vi "Read Directory.vi"(8 "error in (no error)":errorcluster, 11 "TreeDirectory in":refnum<class "TreeDirectoryExt.lvclass">) -> (0 "error out":errorcluster, 2 "Path":path, 3 "TreeDirectory out":refnum<class "TreeDirectoryExt.lvclass">)   [LabVIEW 2026, in "TreeDirectoryExt.lvclass"]
uses:
  TreeDirectoryExt.lvclass
  C:/Program Files/National Instruments/LabVIEW 2026/vi.lib/QSI/QControls/QControl Classes/TreeControl/TreeControl.lvclass
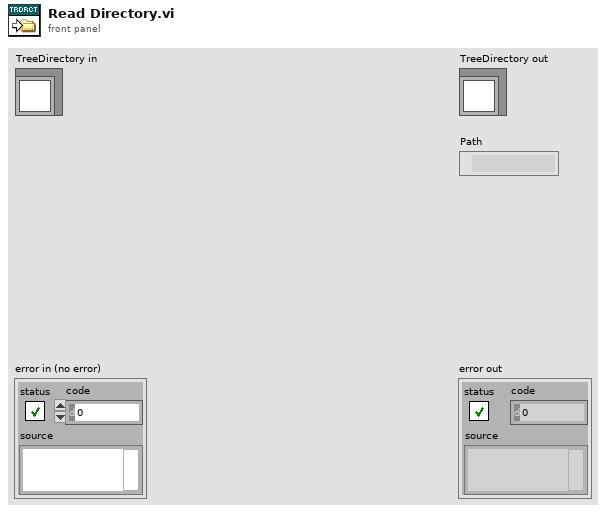
[diagram p1: front panel]
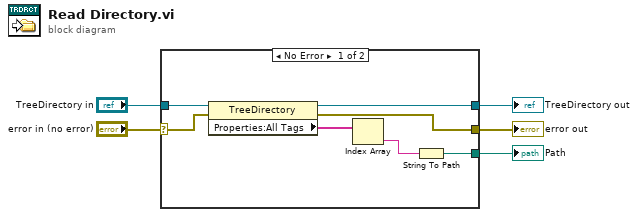
[diagram p0: block diagram]
diagram:
  n1 = case shown="No Error" "error in (no error)" {
    selector: "error in (no error)" -> [w11 w14]
    tunnel: [w6 w14] -> w4
    tunnel: [w9 w13] -> w2
    tunnel: "TreeDirectory in" -> [w12 w13]
    tunnel: [w7 _] -> w1
    frame No Error {
      n2 = property class="TreeDirectory"(reference=w12, error in=w11) -> (reference out=w9:refnum<class "TreeDirectoryExt.lvclass">, error out=w6:errorcluster, "Properties:All Tags"=w10:string[])
      n3 = Index Array(array=w10) -> (element=w8:string)  [unwired: 1 in]
      n4 = String To Path(string=w8) -> (path=w7:path)
    }
    frame Error {
    }
  }
  "error out" <- w4
  "TreeDirectory out" <- w2
  "Path" <- w1
